vi "cylinder.vi"(0 "Cylinder":cluster{"Length":sgl, "Radius":sgl}={"Length"=1.0, "Radius"=1.0}) -> (4 "urdf out":string="<cylinder>\n  <radius>1.00</radius>\n  <length>1.00</length>\n</cylinder>")   [LabVIEW 2012]
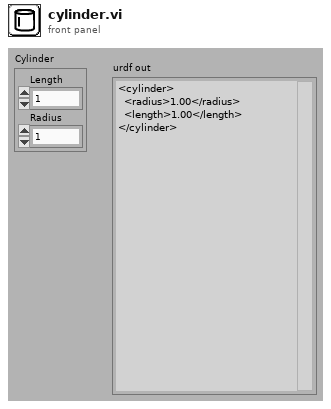
[diagram p1: front panel]
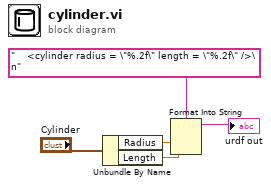
[diagram p0: block diagram]
diagram:
  n1 = Unbundle By Name("Cylinder") -> ("Radius"=w3:sgl, "Length"=w2:sgl)
  n2 = Format Into String(format string="    <cylinder radius = \"%.2f\" length = \"%.2f\" />\n", w3, w2) -> (resulting string=→"urdf out":string)  [unwired: 2 in, 1 out]
